vi "Simple Server - Init.vi"(0 "Process Name for\nthis particular VI":string, 5 "Source":string) -> (4 "Process Variable":string caption="Process Variable Created (Numeric Only)", 15 "error out":errorcluster)   [LabVIEW 2011]
uses:
  <vilib>/variable/tagger/epicsserver/API/internal/List PVs (By Ref).vi
  <vilib>/lvdsc/NI_DSC.lvlib
  <vilib>/variable/tagger/epicsserver/API/NI_EPICS_Server.lvlib
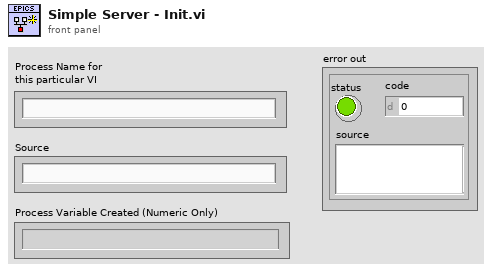
[diagram p1: front panel]
types:
  T1 = enum32{"u32BitField", "bool", "double", "string", "int8", "uint8", "int16", "uint16", "int32", "uint32", "int64", "uint64", "single", "double waveform", "int16 waveform", "array of boolean", "array of int8", "array of uint8", "array of int16", "array of uint16", "array of int32", "array of uint32", "array of int64", "array of uint64", "array of single", "array of double", "array of double waveform", "array of int16 waveform", "array of string", "variant", "timestamp", "fixed point", "custom"}
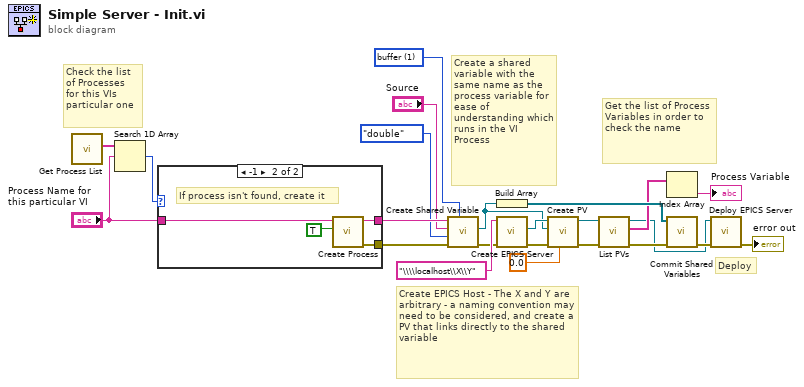
[diagram p0: block diagram]
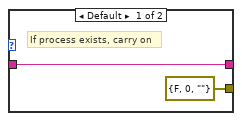
[diagram p2: hidden frame]
diagram:
  w17 = u16 1 items=["commit", "buffer"] ("set mode")
  # "Get the list of Process Variables in order to check the name"
  # "Deploy"
  # "Create a shared variable with the same name as the process variable for ease of understanding which runs in the VI Process"
  # "Create EPICS Host - The X and Y are arbitrary - a naming convention may need to be considered, and create a PV that links directly to the shared variable"
  # "Check the list of Processes for this VIs particular one"
  n1 = call <vilib>:"Get Process List.vi"() -> ("processes"=w20:string[])  [unwired: 10 in, 1 out]
  n2 = Search 1D Array(1D array=w20, element="Process Name for\nthis particular VI") -> (index of element=w21:i32)  [unwired: 1 in]
  n3 = case shown="-1" w21 {
    tunnel: [w25 w28] -> w22
    tunnel: [errorcluster {"status"=FALSE, "code"=0, "source"=""} ("error out") w27] -> w14
    tunnel: "Process Name for\nthis particular VI" -> [w25 w26]
    frame Default {
      # "If process exists, carry on"
    }
    frame -1 {
      # "If process isn't found, create it"
      n4 = call <vilib>:"Create Process.vi"("run?"=TRUE, "process name"=w26) -> ("error out"=w27:errorcluster, "process name out"=w28:string)  [unwired: 8 in]
    }
  }
  n5 = call <vilib>:"Create Shared Variable.vi"("set mode"=w17, "error in (no error)"=w14, "data type"=T1."double", "shared variable name"="Source", "process name"=w22) -> ("error out"=w13:errorcluster, "shared variable"=w9:refnum<k21>)  [unwired: 4 in, 1 out]
  n6 = Build Array(w9) -> (w18:refnum<k21>[])
  n7 = call <vilib>:"Create EPICS Server.vi"("error in (no error)"=w13, "EPICS Server URL in"="\\\\localhost\\X\\Y" ("EPICS Client URL in")) -> ("error out"=w12:errorcluster, "EPICS Server ref"=w11:refnum<data-value>)  [unwired: 7 in, 1 out]
  n8 = call <vilib>:"Create PV.vi"("data type"=0.0, "error in (no error)"=w12, "variable path"=w9, "EPICS Server ref in"=w11) -> ("error out"=w8:errorcluster, "EPICS Server ref out"=w7:refnum<data-value>)  [unwired: 6 in]
  n9 = call-poly <vilib>:"List PVs.vi"("error in (no error)"=w8, "EPICS Server ref in"=w7) -> ("error out"=w4:errorcluster, "PVs"=w6:string[], "EPICS Server ref out"=w1:refnum<data-value>)  [unwired: 7 in]
  n10 = Index Array(array=w6) -> (element=→"Process Variable":string)  [unwired: 1 in]
  n11 = call <vilib>:"Commit Shared Variables.vi"("error in (no error)"=w4, "shared variables"=w18) -> ("error out"=w3:errorcluster)  [unwired: 8 in, 1 out]
  n12 = call <vilib>:"Deploy EPICS Server.vi"("error in (no error)"=w3, "EPICS Server ref in"=w1) -> ("error out"=→"error out":errorcluster)  [unwired: 8 in, 1 out]
